vi "Electrode_selection.vi"(9 "Array of Channel Electrodes":bool[](array[boolean]), 11 "Previous Channel Electrodes":bool[](array[boolean])) -> (3 "Selected Electrode":bool[](array[boolean]), 5 "x != 0?":bool)   [LabVIEW 2014]
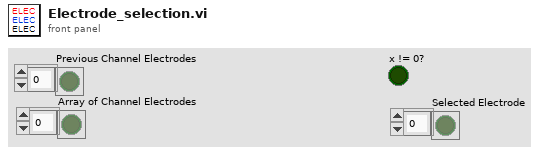
[diagram p1: front panel]
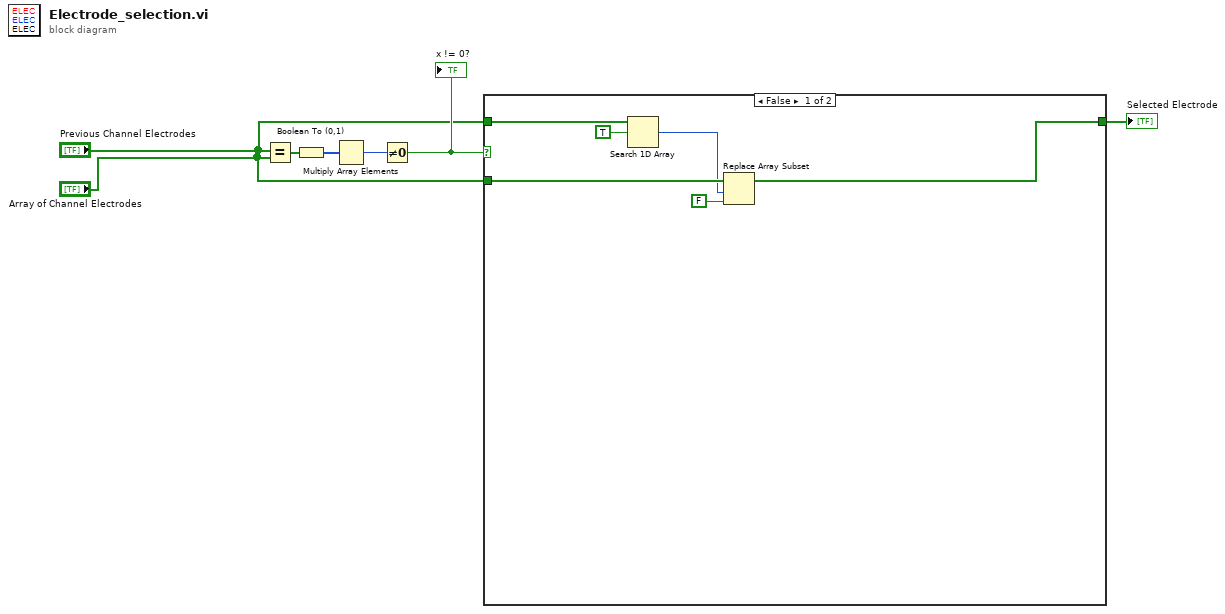
[diagram p0: block diagram]
diagram:
  n1 = Equal?(x="Previous Channel Electrodes", y="Array of Channel Electrodes") -> (x = y?=w7:bool[])
  n2 = Boolean To (0,1)(Boolean=w7) -> (0, 1=w6:i16[])
  n3 = Multiply Array Elements(1:w6) -> (0:w5:i16)
  n4 = Not Equal To 0?(x=w5) -> (x != 0?=w4:bool)
  "x != 0?" <- w4
  n5 = case shown="False" w4 {
    tunnel: "Previous Channel Electrodes" -> [w13 w14]
    tunnel: [w8 w14] -> w2
    tunnel: "Array of Channel Electrodes" -> [w11 _]
    frame False {
      n6 = Search 1D Array(1D array=w13, element=TRUE) -> (index of element=w9:i32)  [unwired: 1 in]
      n7 = Replace Array Subset(array=w11, new element=FALSE ("new element/subarray"), index=w9) -> (w8:bool[])
    }
    frame True {
    }
  }
  "Selected Electrode" <- w2
